vi "DHE_asyncvarsMgr.vi"(7 "action":T2(ring), 8 "error in (no error)":errorcluster, 9 "value":string, 10 "var":string) -> (1 "statusch":bool, 2 "enabled":bool, 3 "names":string[](array[string]))   [LabVIEW 2016]
uses:
  DHE_asyncvarStruct.ctl
panel:
  out "all":bool
  out "vars":T1[](array[typedef])
  in  "var":T1
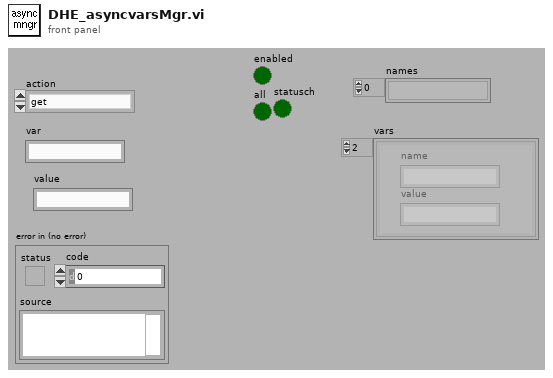
[diagram p1: front panel]
types:
  T1 = typedef "DHE_asyncvarStruct.ctl" = cluster{"name":string, "value":string}
  T2 = enum16{"get", "send", "delete", "add", "clean", "send_all", "send_on", "send_off", "use_stat", "use_async"}
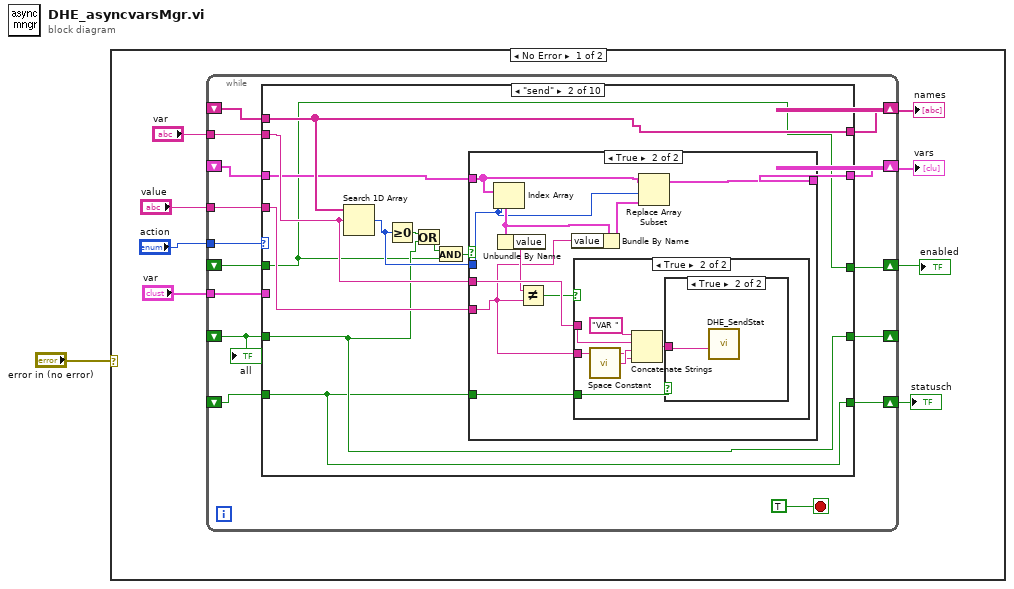
[diagram p0: block diagram]
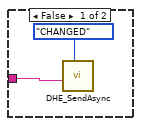
[diagram p5: hidden frame]
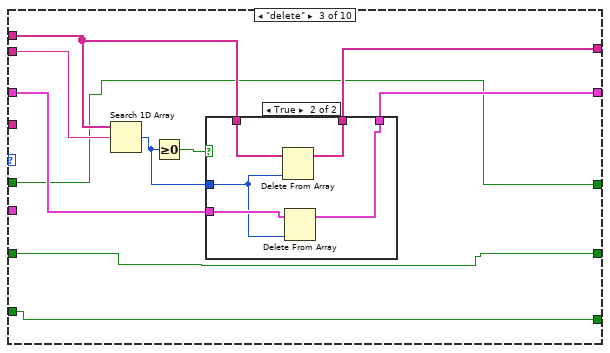
[diagram p6: hidden frame]
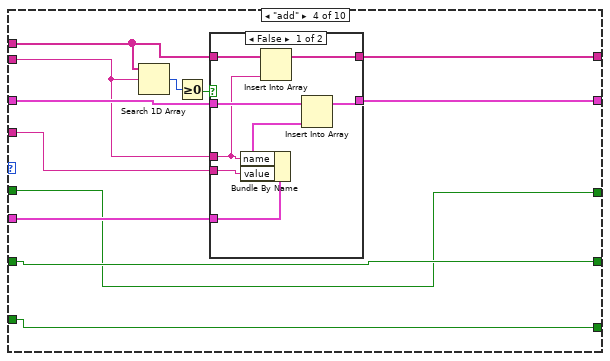
[diagram p8: hidden frame]
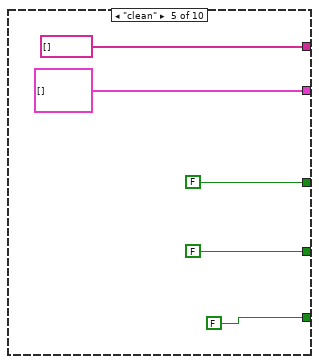
[diagram p10: hidden frame]
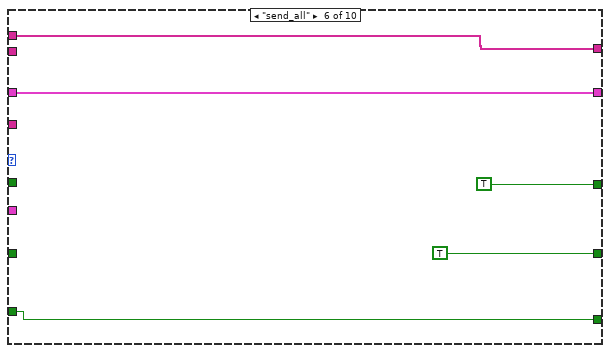
[diagram p11: hidden frame]
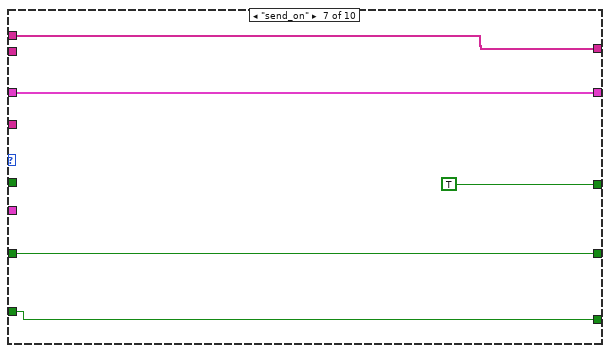
[diagram p12: hidden frame]
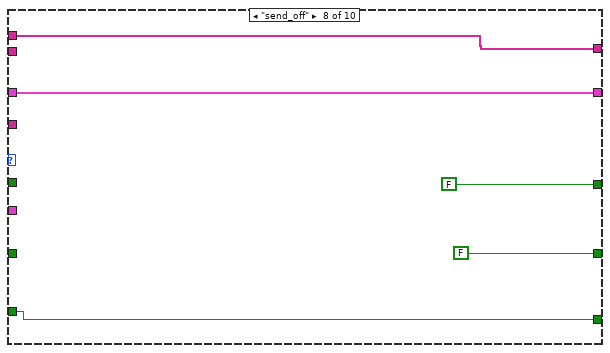
[diagram p13: hidden frame]
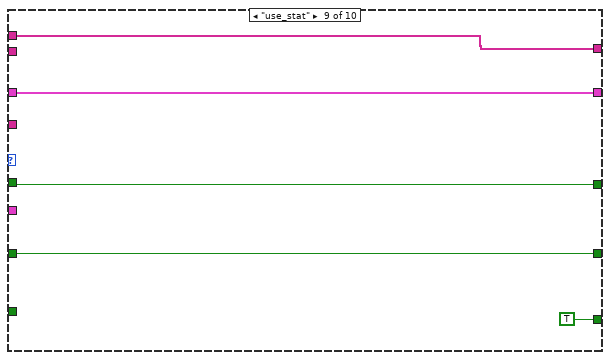
[diagram p14: hidden frame]
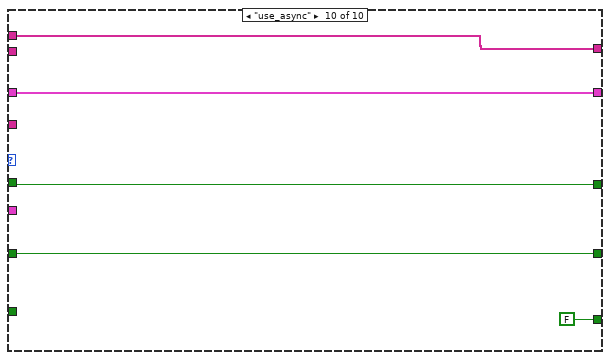
[diagram p15: hidden frame]
diagram:
  n1 = case shown="No Error" "error in (no error)" {
    frame No Error {
      n2 = while {
        tunnel: "action" -> [w23]
        shift-right: [w19] -> w5
        shift-left: _ -> [w18]
        tunnel: "var" -> [w22]
        tunnel: "var" -> [w21]
        tunnel: "value" -> [w20]
        shift-right: [w17] -> w4
        shift-left: _ -> [w16]
        shift-right: [w15] -> _
        shift-left: _ -> [w14]
        shift-right: [w13] -> w2
        shift-left: _ -> [w12]
        shift-right: [w11] -> w3
        shift-left: _ -> [w10]
        stop <- TRUE stop-if-true
        n3 = case shown="\"send\"" w23 {
          tunnel: w22 -> [_ _ _ w90 _ _ _ _ _ _]
          tunnel: w21 -> [_ w39 w65 w82 _ _ _ _ _ _]
          tunnel: w20 -> [_ w38 _ w89 _ _ _ _ _ _]
          tunnel: [w28 w35 w66 w88 T1[] [] w109 w114 w119 w124 w129] -> w19
          tunnel: w18 -> [w28 w36 w69 w87 _ w109 w114 w119 w124 w129]
          tunnel: [w29 w41 w67 w86 string[] [] w110 w115 w120 w125 w130] -> w17
          tunnel: w16 -> [w29 w41 w70 w85 _ w110 w115 w120 w125 w130]
          tunnel: [w27 w34 w64 w81 FALSE TRUE w113 FALSE w122 w127] -> w15
          tunnel: w14 -> [w27 w34 w64 w81 _ _ w113 _ w122 w127]
          tunnel: [w26 w31 w63 w80 FALSE TRUE TRUE FALSE w123 w128] -> w13
          tunnel: w12 -> [w26 w31 w63 w80 _ _ _ _ w123 w128]
          tunnel: [w25 w30 w62 w79 FALSE w106 w111 w116 TRUE FALSE] -> w11
          tunnel: w10 -> [w25 w30 w62 w79 _ w106 w111 w116 _ _]
          frame "get", Default {
          }
          frame "send" {
            n4 = Search 1D Array(1D array=w41, element=w39) -> (index of element=w37:i32)  [unwired: 1 out]
            n5 = Greater Or Equal To 0?(x=w37) -> (x >= 0?=w40:bool)
            n6 = Or(x=w40, y=w34) -> (x .or. y?=w32:bool)
            n7 = And(x=w32, y=w31) -> (x .and. y?=w33:bool)
            n8 = case shown="True" w33 {
              tunnel: w39 -> [_ w47]
              tunnel: w38 -> [_ w45]
              tunnel: w37 -> [_ w49]
              tunnel: w36 -> [w42 w50]
              tunnel: [w42 w48] -> w35
              tunnel: w30 -> [_ w43]
              frame False {
              }
              frame True {
                n9 = Index Array(array=w50, index=w49) -> (element=w52:T1)
                n10 = Unbundle By Name(w52) -> ("value"=w46:string)
                n11 = Not Equal?(x=w46, y=w45) -> (x != y?=w44:bool)
                n12 = Bundle By Name(cluster=w52, "value"=w45) -> (w51:T1)
                n13 = case shown="True" w44 {
                  tunnel: w47 -> [_ w57]
                  tunnel: w45 -> [_ w55]
                  tunnel: w43 -> [_ w53]
                  frame False {
                  }
                  frame True {
                    n14 = call <vilib>:"Space Constant.vi"() -> ("String"=w56:string)
                    n15 = Concatenate Strings("VAR " ("string"), w57, w56, w55) -> (w54:string)
                    n16 = case shown="True" w53 {
                      tunnel: w54 -> [w59 w61]
                      frame False {
                        n17 = call "DHE_SendAsync.vi"("type"=enum16{"ERROR", "WARNING", "INFO", "CHANGED"}."CHANGED", "Message"=w59) -> ()  [unwired: 10 out]
                      }
                      frame True {
                        n18 = call "DHE_SendStat.vi"("Message"=w61) -> ()  [unwired: 11 out]
                      }
                    }
                  }
                }
                n19 = Replace Array Subset(array=w50, new element=w51, index=w49) -> (w48:T1[])
              }
            }
          }
          frame "delete" {
            n20 = Search 1D Array(1D array=w70, element=w65) -> (index of element=w68:i32)  [unwired: 1 out]
            n21 = Greater Or Equal To 0?(x=w68) -> (x >= 0?=w71:bool)
            n22 = case shown="True" w71 {
              tunnel: w70 -> [w73 w78]
              tunnel: w69 -> [w72 w76]
              tunnel: w68 -> [_ w74]
              tunnel: [w73 w77] -> w67
              tunnel: [w72 w75] -> w66
              frame False {
              }
              frame True {
                n23 = Delete From Array(array=w78, index=w74) -> (array with subset deleted=w77:string[])  [unwired: 1 in, 1 out]
                n24 = Delete From Array(array=w76, index=w74) -> (array with subset deleted=w75:T1[])  [unwired: 1 in, 1 out]
              }
            }
          }
          frame "add" {
            n25 = Search 1D Array(1D array=w85, element=w82) -> (index of element=w84:i32)  [unwired: 1 out]
            n26 = Greater Or Equal To 0?(x=w84) -> (x >= 0?=w83:bool)
            n27 = case shown="False" w83 {
              tunnel: w90 -> [w98 _]
              tunnel: w89 -> [w97 _]
              tunnel: [w95 w99] -> w88
              tunnel: w87 -> [w94 w99]
              tunnel: w82 -> [w91 _]
              tunnel: [w93 w100] -> w86
              tunnel: w85 -> [w92 w100]
              frame False {
                n28 = Bundle By Name(cluster=w98, "name"=w91, "value"=w97) -> (w96:T1)
                n29 = Insert Into Array(array=w92, new element=w91) -> (w93:string[])  [unwired: 1 in]
                n30 = Insert Into Array(array=w94, new element=w96) -> (w95:T1[])  [unwired: 1 in]
              }
              frame True {
              }
            }
          }
          frame "clean" {
          }
          frame "send_all" {
          }
          frame "send_on" {
          }
          frame "send_off" {
          }
          frame "use_stat" {
          }
          frame "use_async" {
          }
        }
        "all" <- w14
      }
      "statusch" <- w3
      "enabled" <- w2
      "vars" <- w5
      "names" <- w4
    }
    frame Error {
    }
  }
